vi "Sandbox 6 - Add VI to lvclass.vi"() -> ()   [LabVIEW 2022 SP3]
panel:
  out "Path":path
  out "Name":string
  out "Application:All Libraries in Application Instance 2":string[](array[string])
  out "Application:All Libraries in Application Instance":string[](array[string])
  out "Application:Name 2":string
  out "Application:Name":string
  out "This Application":refnum<vi>
  out "Array":string[](array[string])
  out "New VI Path":path
  out "VI Name (initial)":string
  out "LVClassLibrary Ref":refnum<vi>
  out "error out 2":errorcluster
  out "Class Name":string
  out "error out":errorcluster
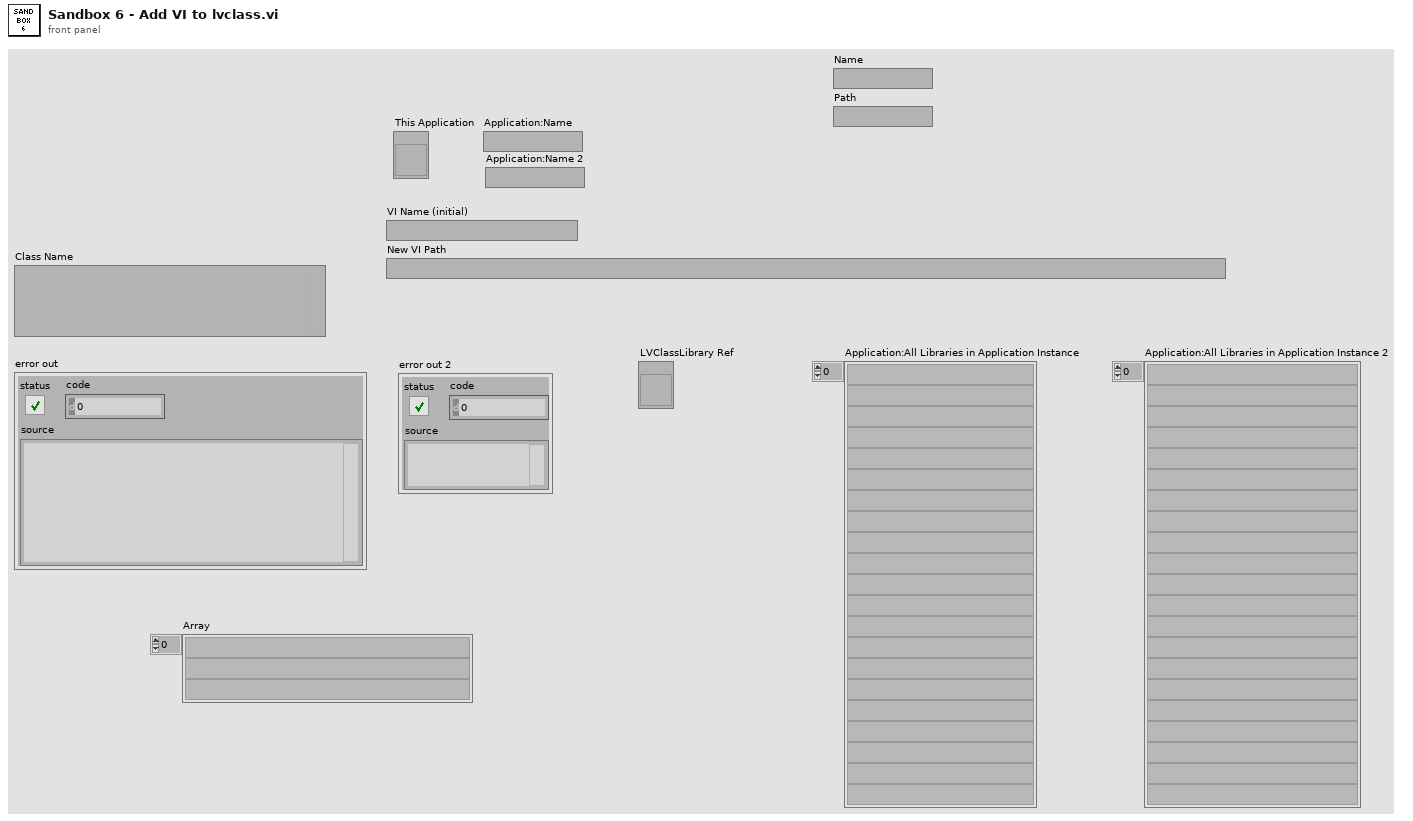
[diagram p1: front panel]
types:
  T1 = enum32{"invalid VI type", "Standard VI", "Control VI", "Global VI", "Polymorphic VI", "Configuration VI", "SubSystem", "Facade VI", "Method VI"}
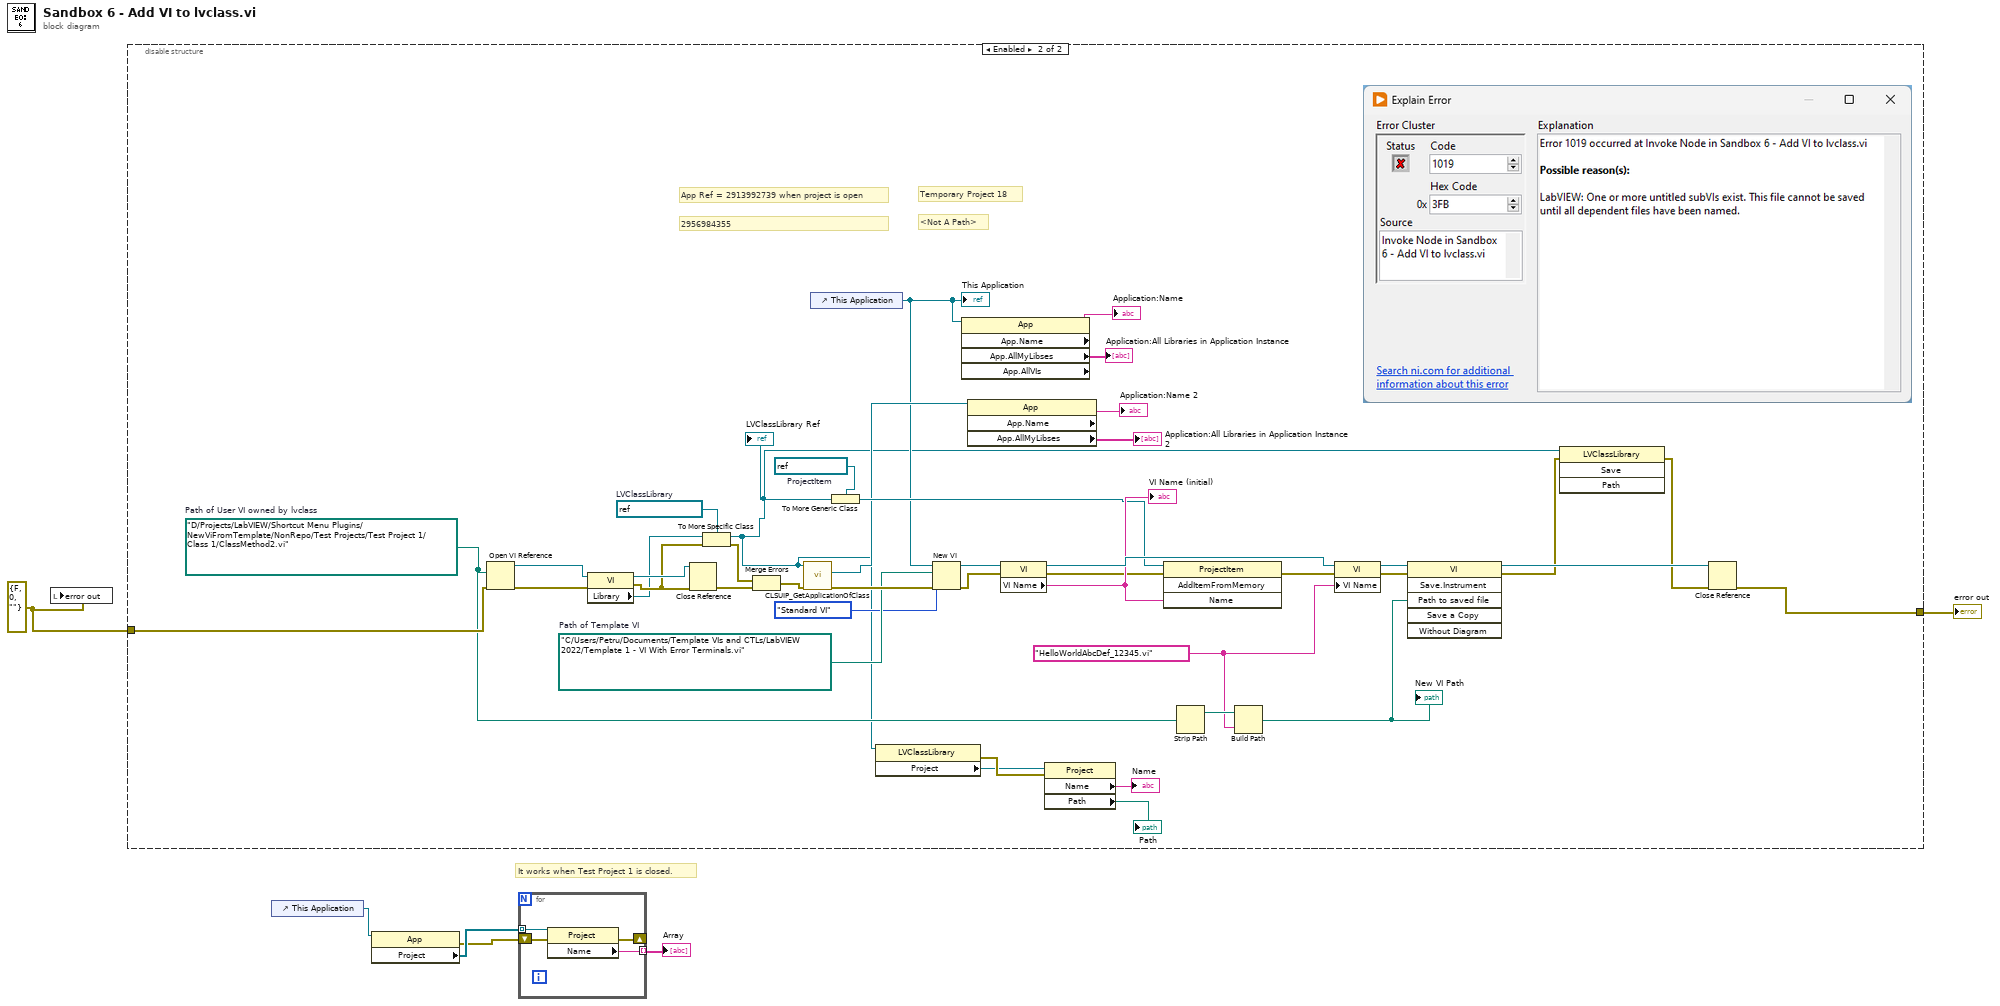
[diagram p0: block diagram]
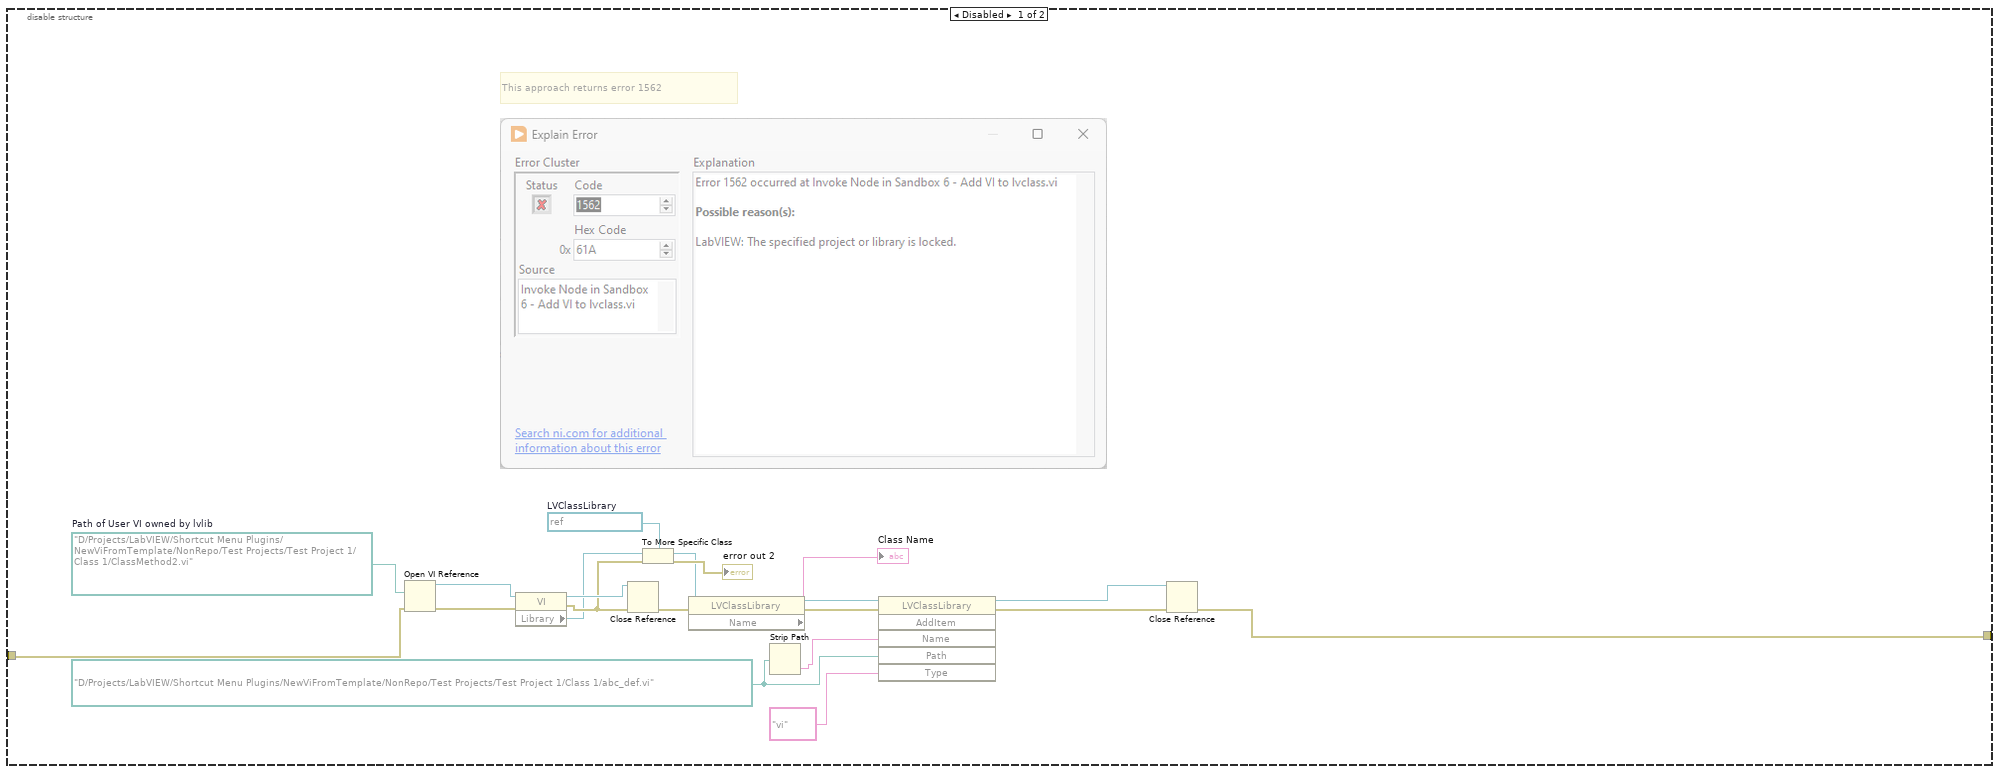
[diagram p2: hidden frame]
diagram:
  w5 = errorcluster {"status"=FALSE, "code"=0, "source"=""} ("error constant")
  # "It works when Test Project 1 is closed."
  n1 = local write "error out"(w5) -> ()
  n2 = disable-structure shown="Enabled" {
    disable-tunnel: [w17 w65] -> w6
    disable-tunnel: w5 -> [w7 w61]
    frame Disabled {
      w15 = refnum<vi> refnum  # LVClassLibrary
      w9 = path "D:/Projects/LabVIEW/Shortcut Menu Plugins/NewViFromTemplate/NonRepo/Test Projects/Test Project 1/Class 1/abc_def.vi"
      w26 = path "D:/Projects/LabVIEW/Shortcut Menu Plugins/NewViFromTemplate/NonRepo/Test Projects/Test Project 1/Class 1/ClassMethod2.vi"  # Path of User VI owned by lvlib
      # "This approach returns error 1562"
      n3 = Open VI Reference(vi path=w26, error in (no error)=w7) -> (vi reference=w24:refnum<vi>, error out=w25:errorcluster)  [unwired: 4 in]
      n4 = property class="VI"(reference=w24, error in=w25) -> (reference out=w18:refnum<vi>, error out=w14:errorcluster, "Library"=w13:refnum<vi>)
      n5 = Close Reference(reference=w18, error in (no error)=w14) -> (error out=w19:errorcluster)
      n6 = To More Specific Class(target class=w15, reference=w13, error in=w14) -> (specific class reference=w11:refnum<vi>, error out=→"error out 2":errorcluster)
      n7 = property class="LVClassLibrary"(reference=w11, error in=w19) -> (reference out=w21:refnum<vi>, error out=w22:errorcluster, "Name"=→"Class Name":string)
      n8 = Strip Path(path=w9) -> (name=w8:string)  [unwired: 1 out]
      n9 = invoke class="LVClassLibrary" method="AddItem"(reference=w21, error in=w22, "Name"=w8, "Path"=w9, "Type"="vi") -> (reference out=w16:refnum<vi>, error out=w23:errorcluster)  [unwired: 1 in, 4 out]
      n10 = Close Reference(reference=w16, error in (no error)=w23) -> (error out=w17:errorcluster)
    }
    frame Enabled {
      w42 = "HelloWorldAbcDef_12345.vi" ("VI Name")
      w49 = refnum<vi> refnum  # ProjectItem
      w53 = path "C:/Users/Petru/Documents/Template VIs and CTLs/LabVIEW 2022/Template 1 - VI With Error Terminals.vi"  # Path of Template VI
      w64 = refnum<vi> refnum  # LVClassLibrary
      w44 = path "D:/Projects/LabVIEW/Shortcut Menu Plugins/NewViFromTemplate/NonRepo/Test Projects/Test Project 1/Class 1/ClassMethod2.vi"  # Path of User VI owned by lvclass
      # "<Not A Path>"
      # "Temporary Project 18"
      # "2956984355"
      # "App Ref = 2913992739 when project is open"
      n11 = Open VI Reference(vi path=w44, error in (no error)=w61) -> (vi reference=w67:refnum<vi>, error out=w68:errorcluster)  [unwired: 4 in]
      n12 = property class="VI"(reference=w67, error in=w68) -> (reference out=w66:refnum<vi>, error out=w63:errorcluster, "Library"=w62:refnum<vi>)
      n13 = Close Reference(reference=w66, error in (no error)=w63) -> (error out=w60:errorcluster)
      n14 = To More Specific Class(target class=w64, reference=w62, error in=w63) -> (specific class reference=w31:refnum<vi>, error out=w58:errorcluster)
      "LVClassLibrary Ref" <- w31
      n15 = Merge Errors(w58, w60) -> (w59:errorcluster)
      n16 = call <resource>:"CLSUIP_GetApplicationOfClass.vi"("error in (no error)"=w59, "LVClassLibrary Ref"=w31) -> ("error out"=w54:errorcluster, "Application"=w36:refnum<vi>)  [unwired: 8 out]
      n17 = control-ref of="This Application"() -> (w32:refnum<vi>)
      "This Application" <- w32
      n18 = To More Generic Class(target class=w49, reference=w31) -> (generic class reference=w48:refnum<vi>)
      n19 = property class="LVClassLibrary"(reference=w31) -> (error out=w30:errorcluster, "Project"=w29:refnum<vi>)  [unwired: 1 in, 1 out]
      n20 = New VI(8:w54, 9:T1."Standard VI" ("vi type (standard vi)"), 10:w53, 11:w32) -> (0:w50:errorcluster, 3:w51:refnum<vi>)  [unwired: 3 out]
      n21 = property class="App" props=["App.Name", "App.AllMyLibses", "App.AllVIs"](reference=w32) -> ("App.Name"=→"Application:Name":string, "App.AllMyLibses"=→"Application:All Libraries in Application Instance":string[])  [unwired: 1 in, 3 out]
      n22 = property class="App"(reference=w36) -> ("App.Name"=→"Application:Name 2":string, "App.AllMyLibses"=→"Application:All Libraries in Application Instance 2":string[])  [unwired: 1 in, 2 out]
      n23 = property class="VI"(reference=w51, error in=w50) -> (reference out=w57:refnum<vi>, error out=w55:errorcluster, "VI Name"=w56:string)
      "VI Name (initial)" <- w56
      n24 = property class="Project"(reference=w29, error in=w30) -> ("Name"=→"Name":string, "Path"=→"Path":path)  [unwired: 2 out]
      n25 = invoke class="ProjectItem" method="AddItemFromMemory"(reference=w48, error in=w55, "Name"=w56) -> (error out=w40:errorcluster)  [unwired: 1 in, 3 out]
      n26 = Strip Path(path=w44) -> (stripped path=w43:path)  [unwired: 1 out]
      n27 = Build Path(base path=w43, name or relative path=w42) -> (appended path=w41:path)
      "New VI Path" <- w41
      n28 = property class="VI"(reference=w57, error in=w40, "VI Name"=w42) -> (reference out=w46:refnum<vi>, error out=w47:errorcluster)
      n29 = invoke class="VI" method="Save.Instrument"(reference=w46, error in=w47, "Path to saved file"=w41) -> (reference out=w45:refnum<vi>, error out=w39:errorcluster)  [unwired: 3 in, 4 out]
      n30 = invoke class="LVClassLibrary" method="Save"(reference=w31, error in=w39) -> (error out=w38:errorcluster)  [unwired: 2 in, 3 out]
      n31 = Close Reference(reference=w45, error in (no error)=w38) -> (error out=w65:errorcluster)
    }
  }
  "error out" <- w6
  n32 = control-ref of="This Application"() -> (w4:refnum<vi>)
  n33 = property class="App"(reference=w4) -> (error out=w2:errorcluster, "Project"=w3:refnum<vi>[])  [unwired: 1 in, 1 out]
  n34 = for {
    shift-right: [w71] -> _
    shift-left: w2 -> [w72]
    tunnel: w3 -> [w70] mode=indexing
    tunnel: [w69] -> w1 mode=indexing
    n35 = property class="Project"(reference=w70, error in=w72) -> (error out=w71:errorcluster, "Name"=w69:string)  [unwired: 1 out]
  }
  "Array" <- w1
